vi "Move relative.vi"(0 "Zaber":T1={"Serial port handle"="", "Axis"="", "Controller #"=0, "Min position"=0.0, "Max position"=0.0, "Min velocity"=0.0, "Max velocity"=0.0, "Firmware"="", "Device ID"=0, "Variable event"=refnum, "Variable ref"=refnum, "Resolution, usteps/step"=0, "Serial port semaphore"=refnum, "Joystick buttons"={"MinDir"=1, "MaxDir"=2, "MedSpeed"=5, "HighSpeed"=6}} {"Joystick buttons"."HighSpeed" min=1 max=25 step=1; "Joystick buttons"."MedSpeed" min=1 max=25 step=1; "Joystick buttons"."MaxDir" min=1 max=25 step=1; "Joystick buttons"."MinDir" min=1 max=25 step=1}, 2 "Distance, mm":dbl, 5 "error in":errorcluster) -> (11 "Start time, ms":u32, 14 "Zaber out":T1={"Serial port handle"="", "Axis"="", "Controller #"=0, "Min position"=0.0, "Max position"=0.0, "Min velocity"=0.0, "Max velocity"=0.0, "Firmware"="", "Device ID"=0, "Variable event"=refnum, "Variable ref"=refnum, "Resolution, usteps/step"=0, "Serial port semaphore"=refnum, "Joystick buttons"={"MinDir"=1, "MaxDir"=2, "MedSpeed"=5, "HighSpeed"=6}} {"Joystick buttons"."HighSpeed" min=1 max=25 step=1; "Joystick buttons"."MedSpeed" min=1 max=25 step=1; "Joystick buttons"."MaxDir" min=1 max=25 step=1; "Joystick buttons"."MinDir" min=1 max=25 step=1}, 16 "Position, mm":dbl, 19 "error out":errorcluster)   [LabVIEW 2018]
uses:
  Zaber.ctl
  GenericDataEvent/GenericEvent.ctl
  ZaberVariables.ctl
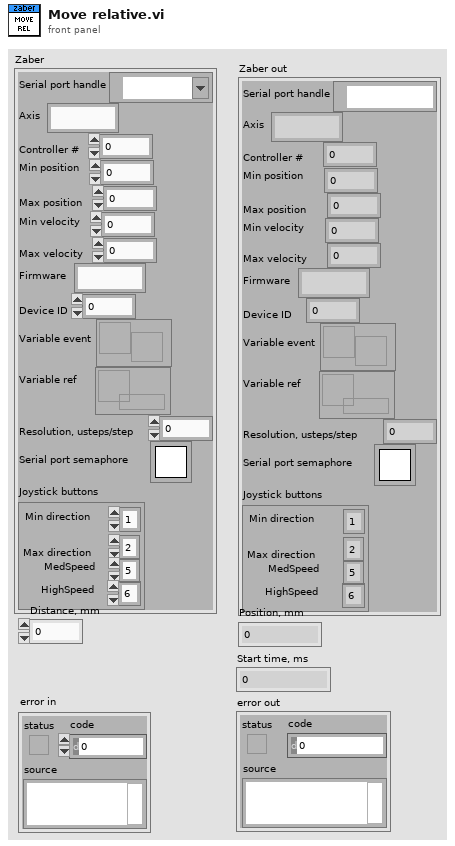
[diagram p1: front panel]
types:
  T1 = typedef "Zaber.ctl" = cluster{"Serial port handle":refnum<visa-resource-name>, "Axis":string, "Controller #":u8, "Min position":dbl, "Max position":dbl, "Min velocity":dbl, "Max velocity":dbl, "Firmware":string, "Device ID":i32, "Variable event":T2, "Variable ref":refnum<data-value>, "Resolution, usteps/step":i32, "Serial port semaphore":T3, "Joystick buttons":cluster{"MinDir":i32, "MaxDir":i32, "MedSpeed":i32, "HighSpeed":i32}}
  T2 = typedef "GenericEvent.ctl" = refnum<user-event>
  T3 = typedef "Semaphore RefNum" = refnum<k1>
  T4 = typedef "ZaberVariables.ctl" = cluster{"Position":i32, "Speed":i32, "Min soft position":dbl, "Max soft position":dbl, "Accelaration":i32}
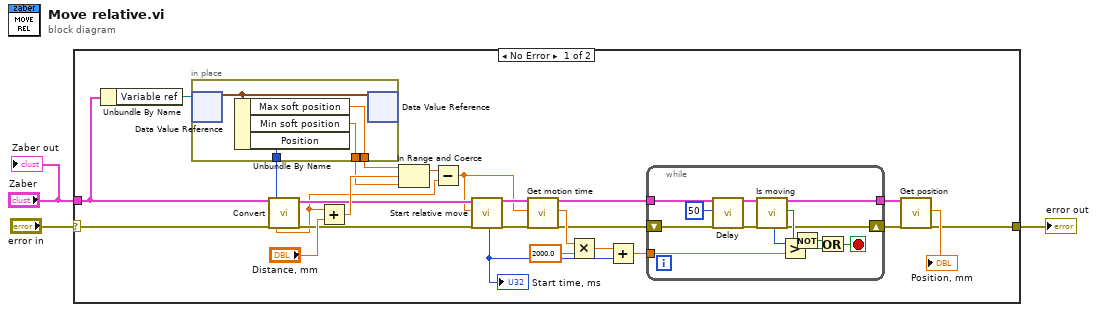
[diagram p0: block diagram]
diagram:
  n1 = case shown="No Error" "error in" {
    selector: "error in" -> [w6 w46]
    tunnel: [w7 w46] -> w2
    tunnel: "Zaber" -> [w12 _]
    frame No Error {
      n2 = Unbundle By Name(w12) -> ("Variable ref"=w15:refnum<data-value>)
      n3 = in-place {
        in-place-border: [w33] -> w8
        in-place-border: [w31] -> w5
        in-place-border: [w30] -> w4
        n4 = in-place-dvr #1(w15) -> (w32:T4)  [unwired: 1 out]
        n5 = Unbundle By Name(w32) -> ("Max soft position"=w31:dbl, "Min soft position"=w30:dbl, "Position"=w33:i32)
        n6 = in-place-dvr #1(w32) -> ()  [unwired: 2 out]
      }
      n7 = call "Convert.vi"("Zaber"=w12, "error in"=w6, "Position, usteps"=w8) -> ("Position, mm"=w11:dbl, "Zaber out"=w14:T1, "error out"=w13:errorcluster)  [unwired: 8 in, 6 out]
      n8 = Add(x=w11, y="Distance, mm") -> (x+y=w23:dbl)
      n9 = In Range and Coerce(upper limit=w5, x=w23, lower limit=w4) -> (coerced(x)=w20:dbl)  [unwired: 1 out]
      n10 = Subtract(x=w20, y=w11) -> (x-y=w10:dbl)
      n11 = call "Start relative move.vi"("Zaber"=w14, "Distance, mm"=w10, "error in"=w13) -> ("Start time, ms"=w21:u32, "Zaber out"=w19:T1, "error out"=w27:errorcluster)  [unwired: 14 in]
      "Start time, ms" <- w21
      n12 = call "Get motion time.vi"("Zaber"=w19, "Distance, mm"=w10, "error in"=w27) -> ("Zaber out"=w26:T1, "Motion time, s"=w25:dbl, "error out"=w18:errorcluster)  [unwired: 14 in]
      n13 = Multiply(x=w25, y=2000.0) -> (x*y=w24:dbl)
      n14 = Add(x=w24, y=w21) -> (x+y=w28:dbl)
      n15 = while {
        tunnel: w26 -> [w34]
        shift-right: [w35] -> w22
        shift-left: w18 -> [w42]
        tunnel: w28 -> [w45]
        tunnel: [w39] -> w17
        stop <- w43 stop-if-true
        n16 = call "Delay.vi"("Delay, ms"=u32 50, "error in"=w42) -> ("error out"=w41:errorcluster)  [unwired: 17 in]
        n17 = call "Is moving.vi"("Zaber"=w34, "error in"=w41) -> ("Command time, ms"=w36:u32, "Zaber out"=w39:T1, "Is moving?"=w38:bool, "error out"=w35:errorcluster)  [unwired: 14 in]
        n18 = Greater?(x=w36, y=w45) -> (0:w44:bool)
        n19 = Not(x=w38) -> (.not. x?=w37:bool)
        n20 = Or(x=w37, y=w44) -> (x .or. y?=w43:bool)
      }
      n21 = call "Get position.vi"("Zaber"=w17, "error in"=w22) -> ("PositionRb"=→"Position, mm":dbl, "error out"=w7:errorcluster)  [unwired: 13 in, 3 out]
    }
    frame Error {
    }
  }
  "error out" <- w2
  "Zaber out" <- "Zaber"
